vi "subSave_PatchParams.vi"(9 "Scaled output":cluster{"xo":i32, dbl, "data":dbl[][]}(graph)={"xo"=0, 5e-05, "data"=array2x40000[80000 elements]}, 10 "Patch quality":T1={"Ra (MΩ)"=236.79401827082728, "Rm (MΩ)"=5201.968657026799, "Cm (pF)"=4.323624616129607, "RC constant (msec)"=1.0238084463479926, "Steady state current (pA)"=9.611745724853648}, 11 "Base path":path=path "C:/Peng/Data/2014-05-13 neuron PZ066 DRH344/DRH344/fov2") -> ()   [LabVIEW 2015]
panel:
  out "Text":string
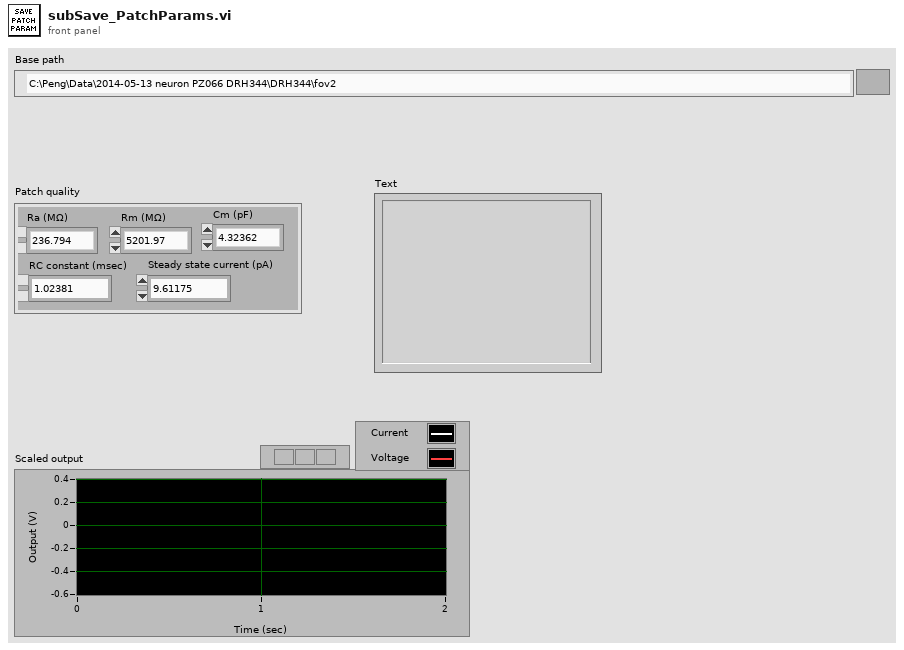
[diagram p1: front panel]
types:
  T1 = cluster{"Ra (MΩ)":dbl, "Rm (MΩ)":dbl, "Cm (pF)":dbl, "RC constant (msec)":dbl, "Steady state current (pA)":dbl}
  T2 = cluster{"Ra (MΩ)":string, "Rm (MΩ)":string, "Cm (pF)":string, "RC constant (msec)":string, "Steady state current (pA)":string}
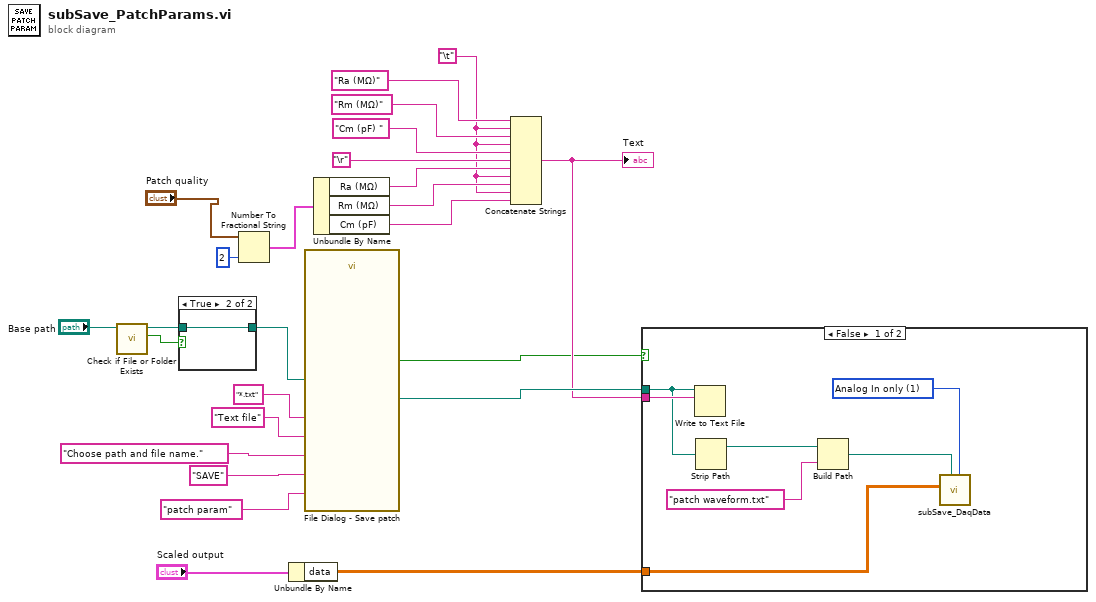
[diagram p0: block diagram]
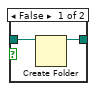
[diagram p3: hidden frame]
diagram:
  w7 = "\t"
  n1 = call <vilib>:"Check if File or Folder Exists.vi"("path"="Base path") -> ("file or folder exists?"=w18:bool, "dup path"=w19:path)  [unwired: 8 in, 1 out]
  n2 = case shown="True" w18 {
    tunnel: w19 -> [w27 w28]
    tunnel: [w26 w28] -> w16
    frame False {
      n3 = Create Folder(path (use dialog)=w27) -> (created path=w26:path)  [unwired: 2 in, 2 out]
    }
    frame True {
    }
  }
  n4 = Number To Fractional String(number="Patch quality", precision (6)=i16 2) -> (F-format string=w2:T2)  [unwired: 2 in]
  n5 = Unbundle By Name("Scaled output") -> ("data"=w4:dbl[][])
  n6 = call "File Dialog - Save patch"("start path"=w16, "prompt"="Choose path and file name.", "button label"="SAVE", "default name"="patch param" ("button label"), "pattern (all files)"="*.txt" ("default name"), "pattern label"="Text file" ("default name")) -> ("selected path"=w20:path, "cancelled"=w6:bool)  [unwired: 6 in, 2 out]
  n7 = Unbundle By Name(w2) -> ("Ra (MΩ)"=w10:string, "Rm (MΩ)"=w9:string, "Cm (pF)"=w8:string)
  n8 = Concatenate Strings("Ra (MΩ)", w7, "Rm (MΩ)", w7, "Cm (pF) ", "\r", w10, w7, w9, w7, w8) -> (w15:string)
  "Text" <- w15
  n9 = case shown="False" w6 {
    tunnel: w20 -> [w34 _]
    tunnel: w15 -> [w35 _]
    tunnel: w4 -> [w31 _]
    frame False {
      w30 = u16 1 items=["Complete waveforms", "Analog In only", "Optopatch"] ("Waveform type")
      n10 = Write to Text File(file (use dialog)=w34, text=w35) -> ()  [unwired: 2 in, 3 out]
      n11 = Strip Path(path=w34) -> (stripped path=w33:path)  [unwired: 1 out]
      n12 = Build Path(base path=w33, name or relative path="patch waveform.txt") -> (appended path=w29:path)
      n13 = call "subSave_DaqData.vi"("Waveform type (complete)"=w30, "path"=w29, "AI waveform"=w31) -> ()  [unwired: 8 in, 1 out]
    }
    frame True {
    }
  }
